vi "Add String with Quote.vi"(5 "Initial String (\"\")":string, 7 "String (\"\")":string, 11 "Error In":errorcluster caption="エラー入力") -> (6 "Resulting String":string, 15 "Error Out":errorcluster caption="エラー出力")   [LabVIEW 2020, in "Yokogawa GX Series.lvlib"]
doc: "Adds quote to string and concatenate to initial string."
uses:
  <instrlib>/Yokogawa GX Series/Yokogawa GX Series.lvlib
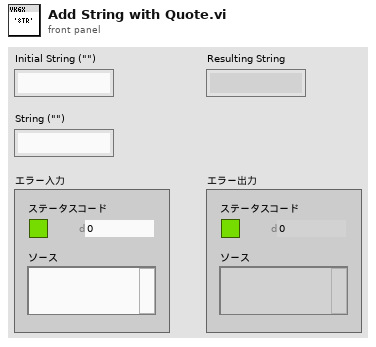
[diagram p1: front panel]
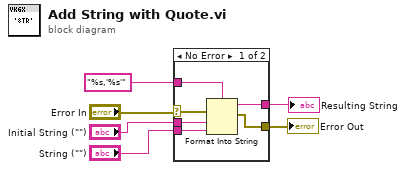
[diagram p0: block diagram]
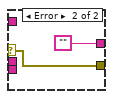
[diagram p2: hidden frame]
diagram:
  n1 = case shown="No Error" "Error In" {
    selector: "Error In" -> [w7 w14]
    tunnel: "%s,'%s'" -> [w12 _]
    tunnel: "Initial String (\"\")" -> [w11 _]
    tunnel: "String (\"\")" -> [w10 _]
    tunnel: [w9 ""] -> w3
    tunnel: [w8 w14] -> w2
    frame No Error {
      n2 = Format Into String(format string=w12, error in=w7, w11, w10) -> (resulting string=w9:string, error out=w8:errorcluster)  [unwired: 1 in]
    }
    frame Error {
    }
  }
  "Resulting String" <- w3
  "Error Out" <- w2
